vi "init_chessboard--set starting square explored.vi"(8 "error in (no error)":errorcluster, 10 "starting_square":T3, 11 "chessboard in":T1[][](array[typedef])) -> (0 "error out":errorcluster, 3 "chessboard out (starting square marked as explored)":T1[][](array[typedef]))   [LabVIEW 2020, in "core.lvlib"]
uses:
  core.lvlib
  core_data/core_data.ctl
  core_data/tour_in_progress.ctl
  core_data/chessboard_index.ctl
  core_data/chess_square.ctl
  core_data/neighbour_square.ctl
  core_data/core_data.lvlib
  PTRL/errors/errors.lvlib
panel:
  out "chess_square":T1
  out "core_data":T4
  # "Development\ncontrols/indicators useful for development and testing, but which are not outputs of the VI"
  # "Input\nInputs to the VI"
  # "Output\nOutputs of the VI"
  # "Description\n\nBlank VI with error handling case. \n\nSummarize the use of this VI in this space."
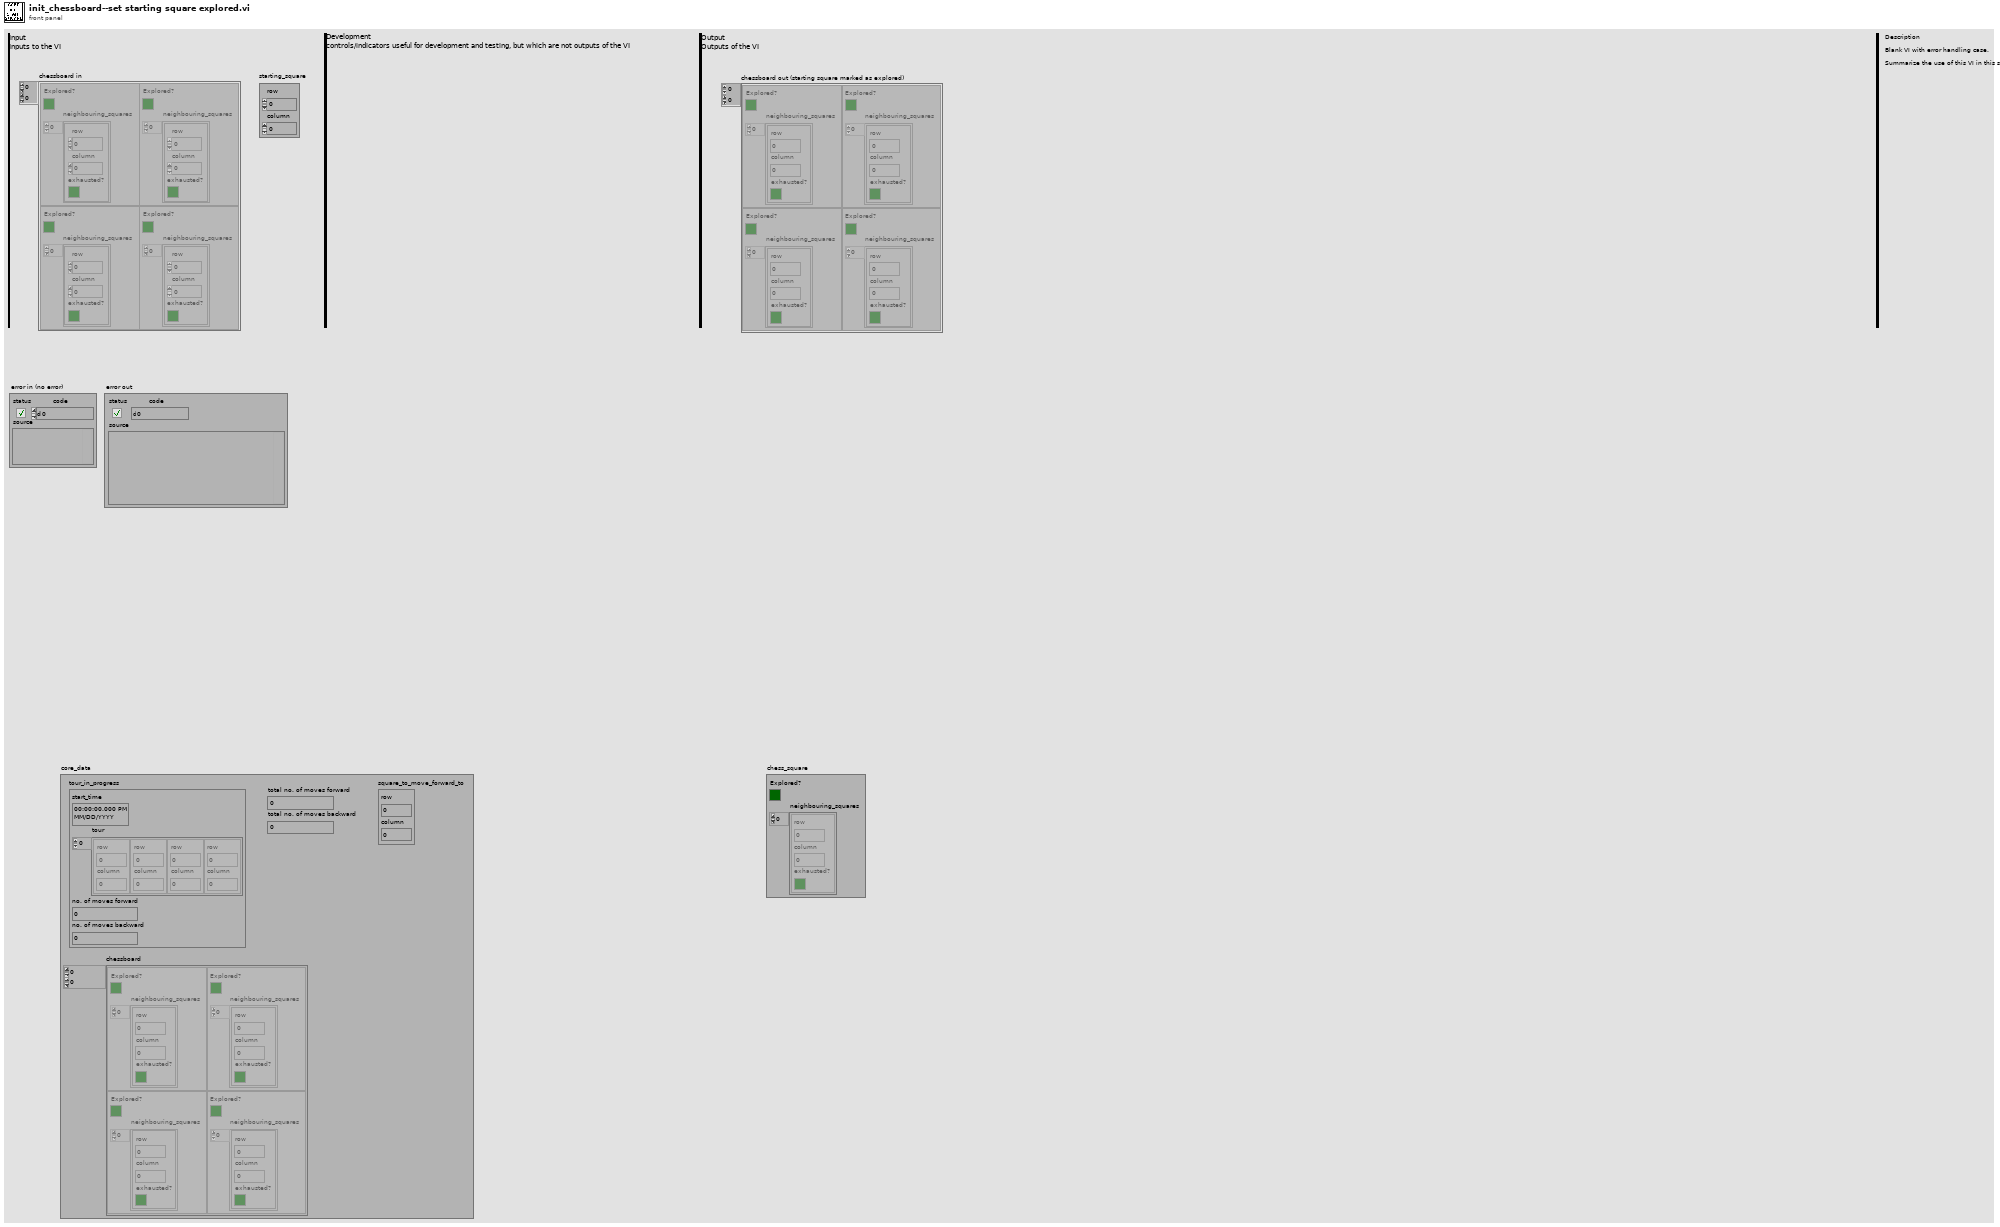
[diagram p1: front panel]
types:
  T1 = typedef "core.lvlib/core_data.lvlib/chess_square.ctl" = cluster{"Explored?":bool, "neighbouring_squares":T2[]}
  T2 = typedef "core.lvlib/core_data.lvlib/neighbour_square.ctl" = cluster{"row":u8, "column":u8, "exhausted?":bool}
  T3 = typedef "core.lvlib/core_data.lvlib/chessboard_index.ctl" = cluster{"row":u8, "column":u8}
  T4 = typedef "core.lvlib/core_data.lvlib/core_data.ctl" = cluster{"tour_in_progress":T5, "total no. of moves forward":u64, "total no. of moves backward":u64, "chessboard":T1[][], "square_to_move_forward_to":T3}
  T5 = typedef "core.lvlib/core_data.lvlib/tour_in_progress.ctl" = cluster{"start_time":timestamp, "tour":T3[], "no. of moves forward":u64, "no. of moves backward":u64}
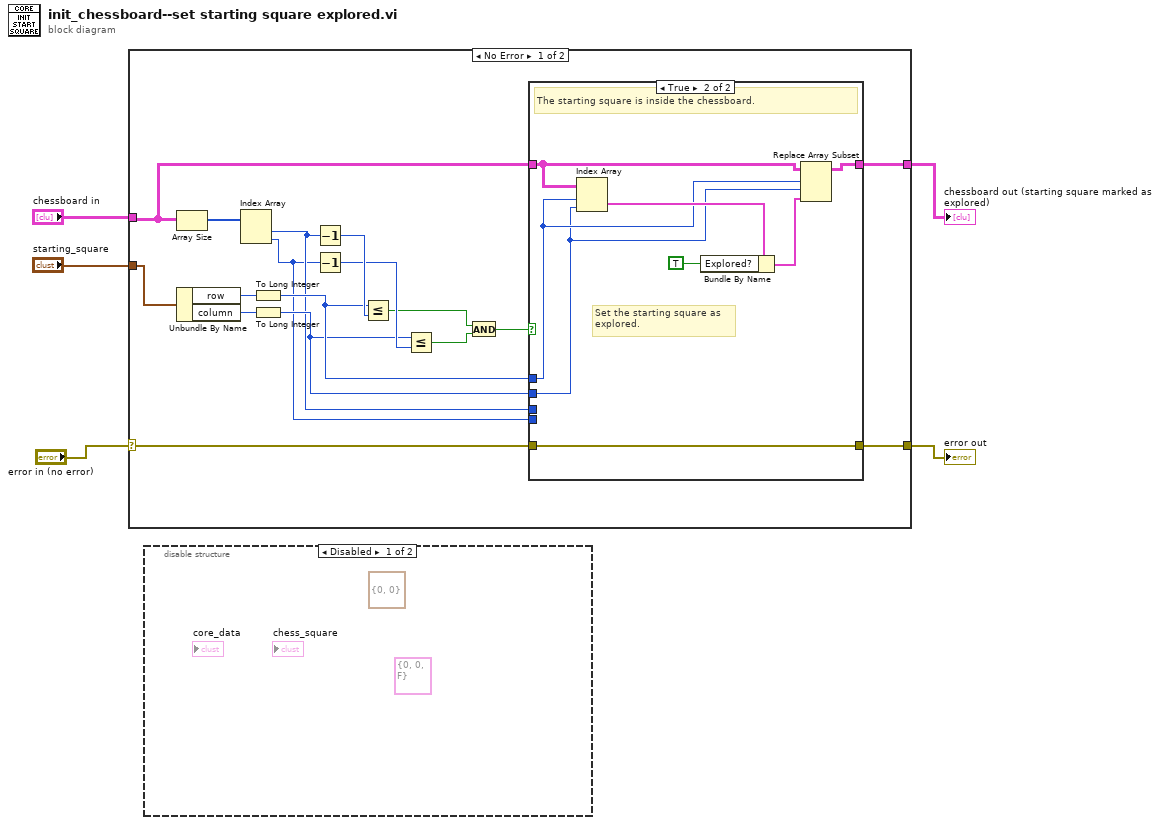
[diagram p0: block diagram]
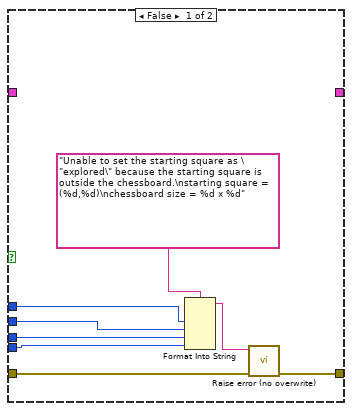
[diagram p2: hidden frame]
diagram:
  n1 = case shown="No Error" "error in (no error)" {
    selector: "error in (no error)" -> [w22 w39]
    tunnel: [w13 w39] -> w4
    tunnel: "chessboard in" -> [w11 _]
    tunnel: "starting_square" -> [w20 _]
    tunnel: [w8 _] -> w1
    frame No Error {
      n2 = Array Size(array=w11) -> (size(s)=w21:i32[])
      n3 = Unbundle By Name(w20) -> ("row"=w19:u8, "column"=w16:u8)
      n4 = Index Array(array=w21) -> (element #1=w7:i32, element #2=w6:i32)  [unwired: 2 in]
      n5 = To Long Integer(number=w19) -> (32bit integer=w10:i32)
      n6 = To Long Integer(number=w16) -> (32bit integer=w9:i32)
      n7 = Decrement(x=w7) -> (x-1=w18:i32)
      n8 = Decrement(x=w6) -> (x-1=w17:i32)
      n9 = Less Or Equal?(x=w10, y=w18) -> (x <= y?=w15:bool)
      n10 = Less Or Equal?(x=w9, y=w17) -> (x <= y?=w14:bool)
      n11 = And(x=w15, y=w14) -> (x .and. y?=w12:bool)
      n12 = case shown="True" w12 {
        tunnel: w22 -> [w30 w36]
        tunnel: [w29 w36] -> w13
        tunnel: w11 -> [_ w35]
        tunnel: w10 -> [w26 w33]
        tunnel: w9 -> [w25 w32]
        tunnel: [_ w31] -> w8
        tunnel: w7 -> [w24 _]
        tunnel: w6 -> [w23 _]
        frame False {
          n13 = Format Into String(format string="Unable to set the starting square as \"explored\" because the starting square is outside the chessboard.\nstarting square = (%d,%d)\nchessboard size = %d x %d", w26, w25, w24, w23) -> (resulting string=w27:string)  [unwired: 2 in, 1 out]
          n14 = call "Raise error (no overwrite).vi"("error in"=w30, "error message (\"\")"=w27) -> ("error out"=w29:errorcluster)  [unwired: 9 in]
        }
        frame True {
          # "Set the starting square as explored."
          # "The starting square is inside the chessboard."
          n15 = Index Array(array=w35, index (row)=w33, index (col)=w32) -> (element=w38:T1)
          n16 = Bundle By Name(cluster=w38, "Explored?"=TRUE) -> (w34:T1)
          n17 = Replace Array Subset(array=w35, new element=w34, index (row)=w33, index (col)=w32) -> (w31:T1[][])
        }
      }
    }
    frame Error {
    }
  }
  "error out" <- w4
  "chessboard out (starting square marked as explored)" <- w1
  n18 = disable-structure shown="Disabled" {
    frame Disabled {
      (unwired) T2 {"row"=0, "column"=0, "exhausted?"=FALSE} ("neighbour_square")
      (unwired) T3 {"row"=0, "column"=0} ("chessboard_index")
    }
    frame Enabled {
    }
  }
